vi "Parsing variable data.vi"(8 "error in (no error)":errorcluster, 10 "data":string[][](array[string]), 11 "SQL Server Info":T2) -> (0 "error out":errorcluster, 3 "appended array":string[](array[string]))   [LabVIEW 2020]
doc: "This subvi parse the database variable nformation to controls\nInput\n1. SQL server info\n2. Error in\nOutput\n1. Array (Parsed Data in cluster format)\n2. Error out"
uses:
  Shared/MySQL/typedefs/mysql_authentication.ctl
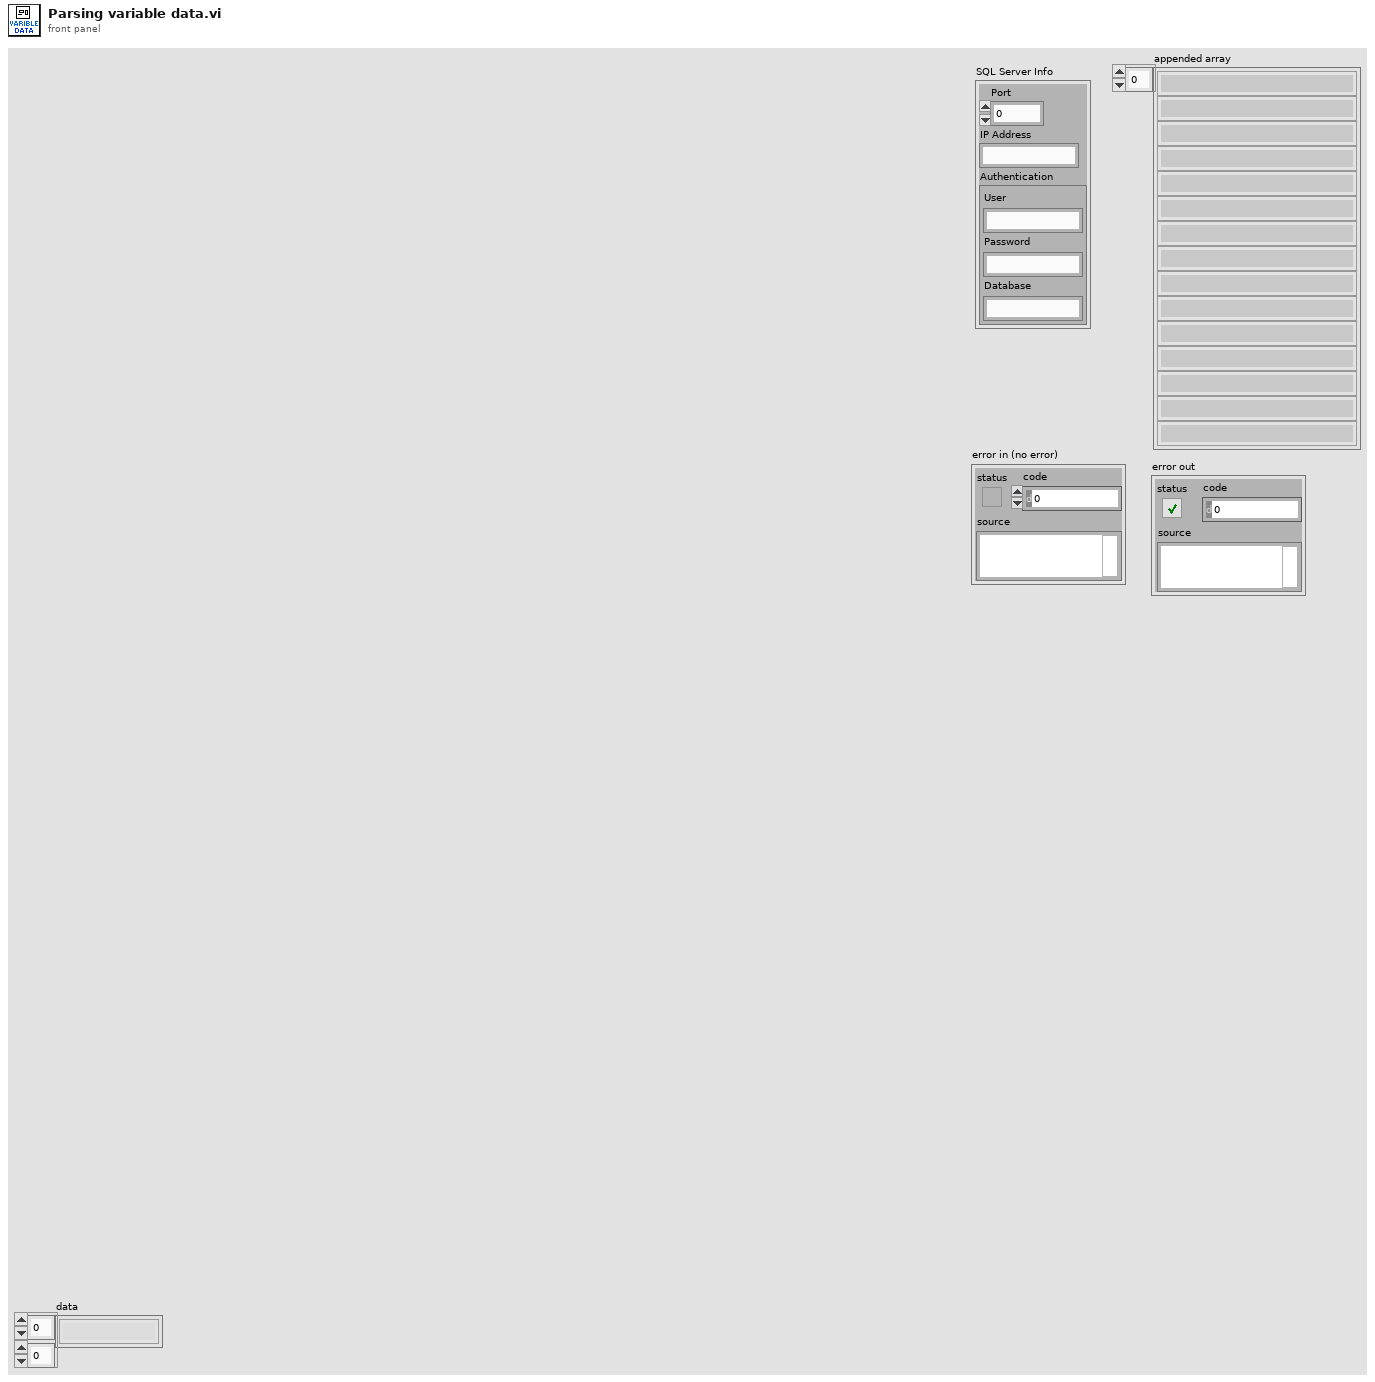
[diagram p1: front panel]
types:
  T1 = typedef "mysql_authentication.ctl" = cluster{"User":string, "Password":string, "Database":string}
  T2 = cluster{"Port":u16, "IP Address":string, "Authentication":T1}
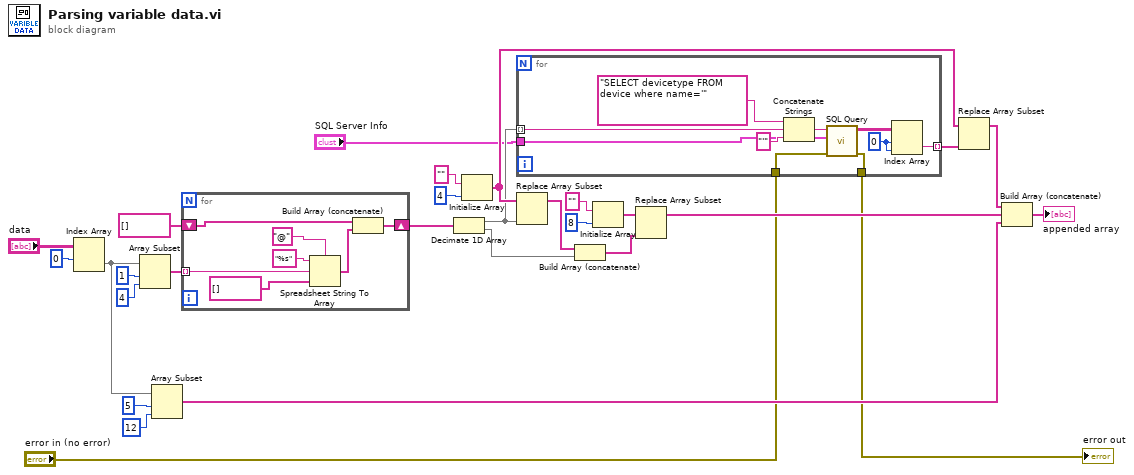
[diagram p0: block diagram]
diagram:
  n1 = Index Array(array="data", index (row)=0) -> (element=w20:string[])  [unwired: 1 in]
  n2 = Array Subset(array=w20, index=1, length=4) -> (w8:string[])
  n3 = Array Subset(array=w20, index=5, length=12) -> (w23:string[])
  n4 = for {
    tunnel: w8 -> [w33] mode=indexing
    shift-right: [w30] -> w12
    shift-left: string[] [] -> [w32]
    n5 = Spreadsheet String To Array(delimiter (Tab)="@", format string="%s", spreadsheet string=w33, array type (2D Dbl)=string[] []) -> (array=w31:string[])
    n6 = Build Array (concatenate)(w32, w31) -> (w30:string[])
  }
  n7 = Decimate 1D Array(w12) -> (w25:string[], w18:string[])
  n8 = Initialize Array("", 4 ("dimension size")) -> (w26:string[])
  n9 = for {
    tunnel: "SQL Server Info" -> [w38]
    tunnel: w25 -> [w42] mode=indexing
    tunnel: [w39] -> w27 mode=indexing
    tunnel: "error in (no error)" -> [w37]
    tunnel: [w36] -> w1
    w40 = 0 ("index (row)")
    n10 = Concatenate Strings("SELECT devicetype FROM device where name='" ("Query"), w42, "'" ("string")) -> (w43:string)
    n11 = call "SQL Query.vi"("error in (no error)"=w37, "SQL Server Info"=w38, "Query"=w43) -> ("error out"=w36:errorcluster, "data"=w41:string[][])  [unwired: 7 in]
    n12 = Index Array(array=w41, index (row)=w40, index (col)=w40) -> (element=w39:string)
  }
  "error out" <- w1
  n13 = Replace Array Subset(array=w26, new element=w25) -> (w17:string[])  [unwired: 1 in]
  n14 = Build Array (concatenate)(w17, w18) -> (w13:string[])
  n15 = Initialize Array("", 8 ("dimension size")) -> (w14:string[])
  n16 = Replace Array Subset(array=w14, new element=w13) -> (w19:string[])  [unwired: 1 in]
  n17 = Replace Array Subset(array=w26, new element=w27) -> (w28:string[])  [unwired: 1 in]
  n18 = Build Array (concatenate)(w28, w19, w23) -> (→"appended array":string[])
